vi "Create New XML File.vi"(8 "error in (no error)":errorcluster, 10 "Output File Folder":path, 11 "XML Handler in":refnum<class "XML Handler.lvclass">) -> (0 "error out":errorcluster, 3 "XML Handler out":refnum<class "XML Handler.lvclass">)   [LabVIEW 2020, in "XML Handler.lvclass"]
uses:
  XML Handler.lvclass
  XML Handler.lvclass/XML Handler.ctl
  <vilib>/xml/Load XML File.vi
  <vilib>/xml/Close Reference(Node).vi
  <vilib>/xml/NI_XML.lvlib
  <resource>/objmgr/DOMUserDefRef.rc
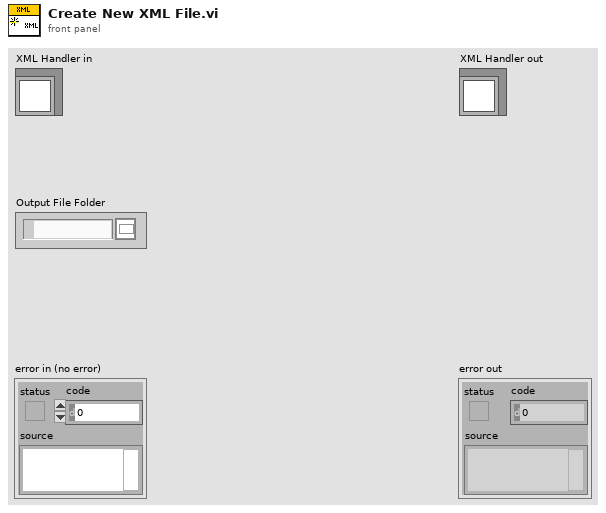
[diagram p1: front panel]
types:
  T1 = enum16{"open", "replace", "create", "open or create", "replace or create", "replace or create with confirmation"}
  T2 = enum32{"invalid app kind", "Development System", "Run Time System", "Student Edition", "Embedded LabVIEW", "Evaluation", "Custom"}
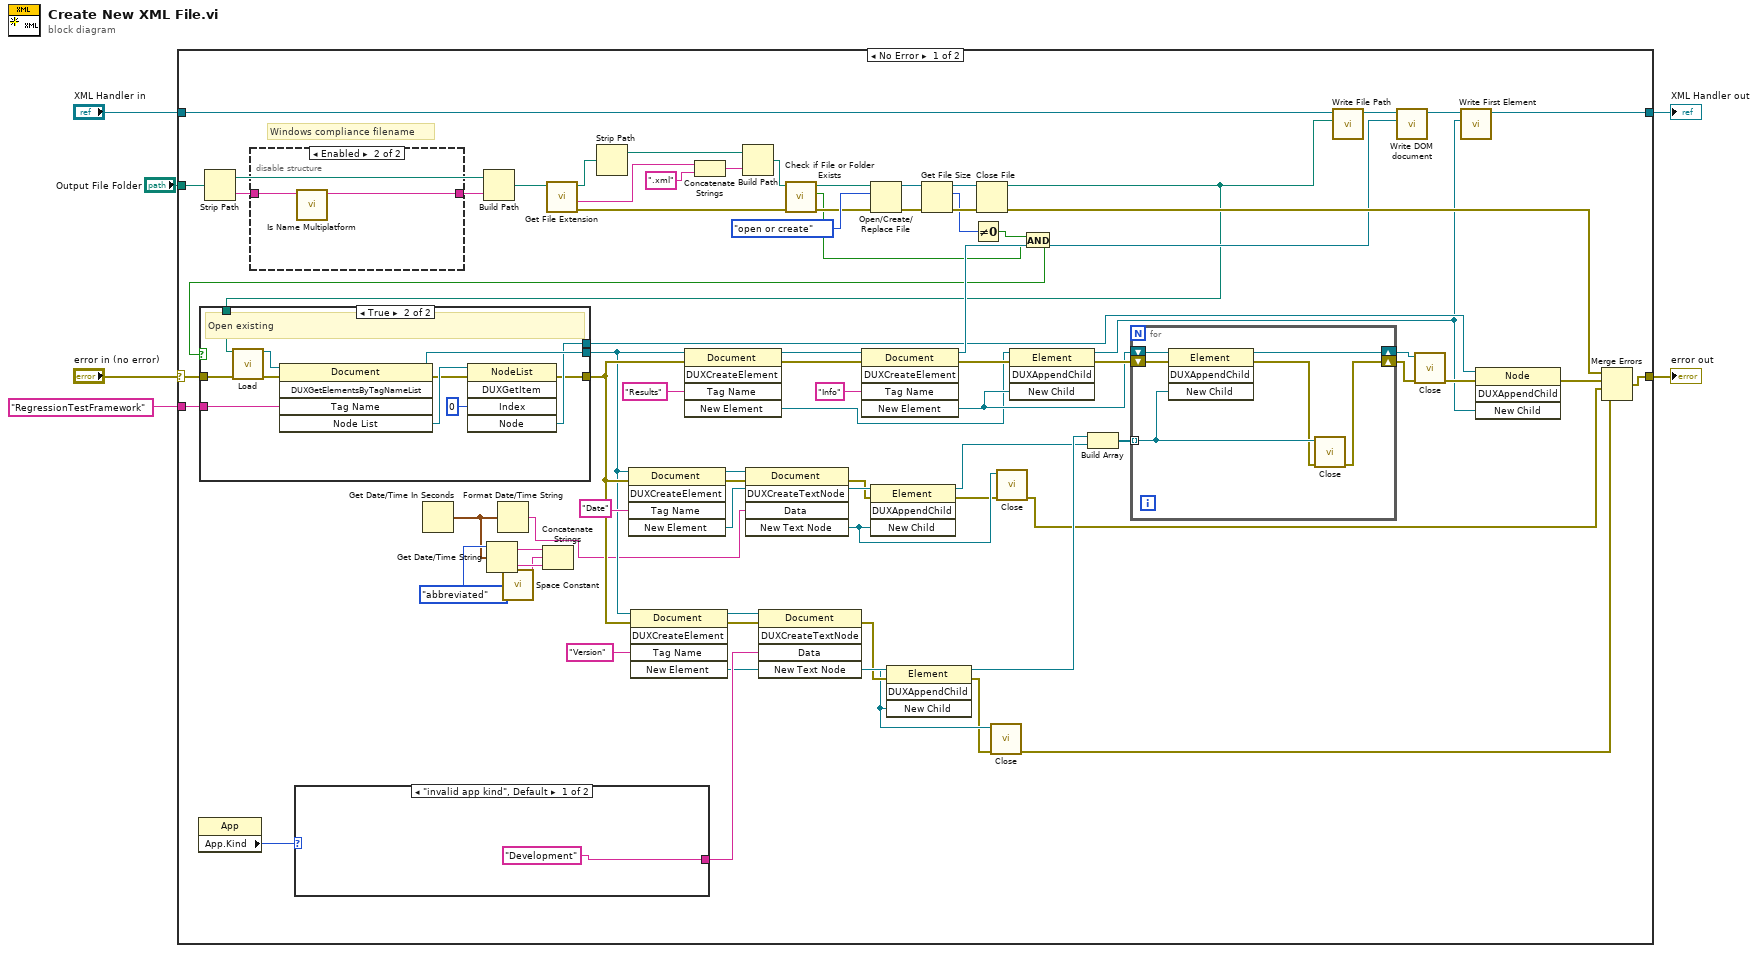
[diagram p0: block diagram]
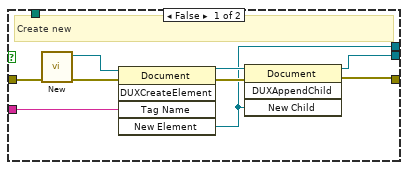
[diagram p2: hidden frame]
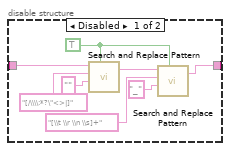
[diagram p3: hidden frame]
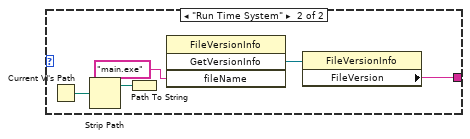
[diagram p4: hidden frame]
diagram:
  n1 = case shown="No Error" "error in (no error)" {
    selector: "error in (no error)" -> [w82 w126]
    tunnel: [w56 w126] -> w5
    tunnel: [w73 w125] -> w3
    tunnel: "XML Handler in" -> [w74 w125]
    tunnel: "Output File Folder" -> [w58 _]
    tunnel: "RegressionTestFramework" ("Tag Name") -> [w23 _]
    frame No Error {
      # "Windows compliance filename"
      n2 = property class="App"() -> ("App.Kind"=w70:T2)  [unwired: 2 in, 2 out]
      n3 = Strip Path(path=w58) -> (stripped path=w59:path, name=w61:string)
      n4 = disable-structure shown="Enabled" {
        disable-tunnel: w61 -> [w110 w118]
        disable-tunnel: [w109 w117] -> w60
        frame Disabled {
          w113 = TRUE ("replace all? (F)")
          n5 = call <vilib>:"Search and Replace Pattern.vi"("string"=w110, "regular expression (\"\")"="[/\\\\:*?\"<>|]" ("regular expression (\"\")"), "replace string (\"\")"="" ("replace string (\"\")"), "replace all? (F)"=w113) -> ("result string"=w114:string)  [unwired: 1 in, 1 out]
          n6 = call <vilib>:"Search and Replace Pattern.vi"("string"=w114, "regular expression (\"\")"="[\\t \\r \\n \\s]+" ("regular expression (\"\") 2"), "replace string (\"\")"="_" ("replace string (\"\") 2"), "replace all? (F)"=w113) -> ("result string"=w109:string)  [unwired: 1 in, 1 out]
        }
        frame Enabled {
          n7 = call <vilib>:"Is Name Multiplatform.vi"("filename"=w118) -> ("suggested filename"=w117:string)  [unwired: 6 in, 4 out]
        }
      }
      n8 = case shown="\"invalid app kind\", Default" w70 {
        tunnel: ["Development" w122] -> w69
        frame "invalid app kind", Default {
        }
        frame "Run Time System" {
          n9 = Current VI's Path() -> (path=w124:path)
          n10 = Strip Path(path=w124) -> (stripped path=w121:path)  [unwired: 1 out]
          n11 = Path To String(path=w121) -> ()  [unwired: 1 out]
          n12 = invoke class="FileVersionInfo" method="GetVersionInfo"("fileName"="main.exe") -> ("GetVersionInfo"=w123:refnum<k24>)  [unwired: 3 in, 3 out]
          n13 = property class="FileVersionInfo"(reference=w123) -> ("FileVersion"=w122:string)  [unwired: 1 in, 2 out]
        }
      }
      n14 = Get Date/Time In Seconds() -> (seconds since 1Jan1904=w62:timestamp)
      n15 = Build Path(base path=w59, name or relative path=w60) -> (appended path=w50:path)
      n16 = Get Date/Time String(date format (0)=enum16{"short", "long", "abbreviated"}."abbreviated", seconds (now)=w62) -> (date string=w79:string, time string=w78:string)  [unwired: 1 in]
      n17 = Format Date/Time String(seconds (now)=w62) -> (date/time string=w7:string)  [unwired: 2 in]
      n18 = call <vilib>:"Space Constant.vi"() -> ("String"=w77:string)
      n19 = Concatenate Strings(w79, w77, w78) -> ()  [unwired: 1 out]
      n20 = call <vilib>:"Get File Extension.vi"("file"=w50) -> ("error out"=w28:errorcluster, "filename without extension"=w51:string, "dup file"=w52:path)  [unwired: 6 in, 2 out]
      n21 = Strip Path(path=w52) -> (stripped path=w54:path)  [unwired: 1 out]
      n22 = Concatenate Strings(w51, ".xml" ("string")) -> (w53:string)
      n23 = Build Path(base path=w54, name or relative path=w53) -> (appended path=w25:path)
      n24 = call <vilib>:"Check if File or Folder Exists.vi"("error in (no error)"=w28, "path"=w25) -> ("error out"=w27:errorcluster, "file or folder exists?"=w11:bool, "dup path"=w26:path)  [unwired: 7 in]
      n25 = Open/Create/Replace File(file path (use dialog)=w26, error in=w27, operation (0:open)=T1."open or create") -> (refnum out=w16:refnum<file>, error out=w17:errorcluster)  [unwired: 3 in, 1 out]
      n26 = Get File Size(file=w16, error in=w17) -> (refnum out=w14:refnum<file>, size (in bytes)=w13:i64, 0:w15:errorcluster)
      n27 = Not Equal To 0?(x=w13) -> (x != 0?=w12:bool)
      n28 = Close File(refnum=w14, error in=w15) -> (path=w24:path, error out=w57:errorcluster)
      n29 = And(x=w12, y=w11) -> (x .and. y?=w10:bool)
      n30 = case shown="True" w10 {
        tunnel: w82 -> [w91 w102]
        tunnel: [w85 w97] -> w21
        tunnel: [w84 w92] -> w22
        tunnel: w24 -> [_ w101]
        tunnel: w23 -> [w88 w99]
        tunnel: [w83 w95] -> w20
        frame False {
          # "Create new"
          n31 = call <vilib>:"New.vi"("error in (no error)"=w91) -> ("error out"=w89:errorcluster, "DOM document out"=w90:refnum<k20>)  [unwired: 7 in]
          n32 = invoke class="Document" method="DUXCreateElement"(reference=w90, error in=w89, "Tag Name"=w88) -> (reference out=w87:refnum<k20>, error out=w86:errorcluster, "New Element"=w83:refnum<k20>)  [unwired: 2 in, 2 out]
          n33 = invoke class="Document" method="DUXAppendChild"(reference=w87, error in=w86, "New Child"=w83) -> (reference out=w85:refnum<k20>, error out=w84:errorcluster)  [unwired: 1 in, 2 out]
        }
        frame True {
          # "Open existing"
          n34 = call-poly <vilib>:"Load.vi"("path to XML document"=w101, "error in (no error)"=w102) -> ("DOM document out"=w100:refnum<k20>, "error out"=w98:errorcluster)  [unwired: 11 in, 1 out]
          n35 = invoke class="Document" method="DUXGetElementsByTagNameList"(reference=w100, error in=w98, "Tag Name"=w99) -> (reference out=w97:refnum<k20>, error out=w93:errorcluster, "Node List"=w96:refnum<k20>)  [unwired: 2 in, 2 out]
          n36 = invoke class="NodeList" method="DUXGetItem"(reference=w96, error in=w93, "Index"=0) -> (error out=w92:errorcluster, "Node"=w95:refnum<k20>)  [unwired: 2 in, 3 out]
        }
      }
      n37 = invoke class="Document" method="DUXCreateElement"(reference=w21, error in=w22, "Tag Name"="Date") -> (reference out=w46:refnum<k20>, error out=w45:errorcluster, "New Element"=w80:refnum<k20>)  [unwired: 2 in, 2 out]
      n38 = invoke class="Document" method="DUXCreateElement"(reference=w21, error in=w22, "Tag Name"="Version") -> (reference out=w44:refnum<k20>, error out=w71:errorcluster, "New Element"=w68:refnum<k20>)  [unwired: 2 in, 2 out]
      n39 = invoke class="Document" method="DUXCreateElement"(reference=w21, error in=w22, "Tag Name"="Results") -> (reference out=w41:refnum<k20>, error out=w40:errorcluster, "New Element"=w19:refnum<k20>)  [unwired: 2 in, 2 out]
      n40 = invoke class="Document" method="DUXCreateTextNode"(reference=w46, error in=w45, "Data"=w7) -> (error out=w43:errorcluster, "New Text Node"=w37:refnum<k20>)  [unwired: 2 in, 3 out]
      n41 = invoke class="Document" method="DUXCreateTextNode"(reference=w44, error in=w71, "Data"=w69) -> (error out=w67:errorcluster, "New Text Node"=w66:refnum<k20>)  [unwired: 2 in, 3 out]
      n42 = invoke class="Document" method="DUXCreateElement"(reference=w41, error in=w40, "Tag Name"="Info") -> (reference out=w31:refnum<k20>, error out=w39:errorcluster, "New Element"=w35:refnum<k20>)  [unwired: 2 in, 2 out]
      n43 = invoke class="Element" method="DUXAppendChild"(reference=w80, error in=w43, "New Child"=w37) -> (reference out=w48:refnum<k20>, error out=w36:errorcluster)  [unwired: 1 in, 2 out]
      n44 = invoke class="Element" method="DUXAppendChild"(reference=w68, error in=w67, "New Child"=w66) -> (reference out=w49:refnum<k20>, error out=w65:errorcluster)  [unwired: 1 in, 2 out]
      n45 = call-poly <vilib>:"Close.vi"("error in (no error)"=w65, "node"=w66) -> ("error out"=w8:errorcluster)  [unwired: 7 in]
      n46 = call-poly <vilib>:"Close.vi"("error in (no error)"=w36, "node"=w37) -> ("error out"=w9:errorcluster)  [unwired: 7 in]
      n47 = invoke class="Element" method="DUXAppendChild"(reference=w19, error in=w39, "New Child"=w35) -> (reference out=w18:refnum<k20>, error out=w38:errorcluster)  [unwired: 1 in, 2 out]
      n48 = Build Array(w49, w48) -> (w47:refnum<k20>[])
      n49 = for {
        shift-right: [w106] -> w30
        shift-left: w35 -> [w107]
        tunnel: w47 -> [w105] mode=indexing
        shift-right: [w103] -> w34
        shift-left: w38 -> [w108]
        n50 = invoke class="Element" method="DUXAppendChild"(reference=w107, error in=w108, "New Child"=w105) -> (reference out=w106:refnum<k20>, error out=w104:errorcluster)  [unwired: 1 in, 2 out]
        n51 = call-poly <vilib>:"Close.vi"("error in (no error)"=w104, "node"=w105) -> ("error out"=w103:errorcluster)  [unwired: 7 in]
      }
      n52 = call "Write File Path.vi"("File Path"=w24, "XML Handler in"=w74) -> ("XML Handler out"=w76:refnum<class "XML Handler.lvclass">)  [unwired: 9 in]
      n53 = call "Write DOM document.vi"("DOM document"=w31, "XML Handler in"=w76) -> ("XML Handler out"=w75:refnum<class "XML Handler.lvclass">)  [unwired: 9 in]
      n54 = call-poly <vilib>:"Close.vi"("error in (no error)"=w34, "node"=w30) -> ("error out"=w33:errorcluster)  [unwired: 7 in]
      n55 = call "Write First Element.vi"("First Element"=w18, "XML Handler in"=w75) -> ("XML Handler out"=w73:refnum<class "XML Handler.lvclass">)  [unwired: 9 in]
      n56 = invoke class="Node" method="DUXAppendChild"(reference=w20, error in=w33, "New Child"=w18) -> (error out=w32:errorcluster)  [unwired: 1 in, 3 out]
      n57 = Merge Errors(w57, w32, w9, w8) -> (w56:errorcluster)
    }
    frame Error {
    }
  }
  "error out" <- w5
  "XML Handler out" <- w3
